vi "Close.vi"(8 "error in (no error)":errorcluster, 11 "SOL Camera in":refnum<class "PL SOL Instruments Camera.lvclass">) -> (0 "error out":errorcluster)   [LabVIEW 2015, in "PL SOL Instruments Camera.lvclass"]
doc: "Closes connection to device."
uses:
  PL SOL Instruments Camera.lvclass
  PL SOL Instruments Camera.lvclass/PL SOL Instruments Camera.ctl
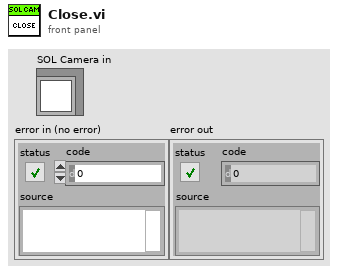
[diagram p1: front panel]
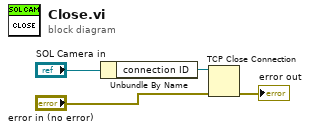
[diagram p0: block diagram]
diagram:
  n1 = Unbundle By Name("SOL Camera in") -> ("connection ID"=w3:refnum<k5>)
  n2 = TCP Close Connection(connection ID=w3, error in (no error)="error in (no error)") -> (error out=→"error out":errorcluster)  [unwired: 1 in, 1 out]
